vi "AB_1000_1100_Project_Build_Info.vi"(7 "action":T1, 8 "error in (no error)":errorcluster, 10 "buildInfo in":T2, 11 "Object In":T3) -> (0 "error out":errorcluster, 2 "buildInfo out":T2, 3 "Object Out":T3)   [LabVIEW 2020]
uses:
  <vilib>/AppBuilder/RW_Project/AB_RW_Project_PropBag_Action.ctl
  <resource>/Framework/Providers/API/ItemRef.ctl
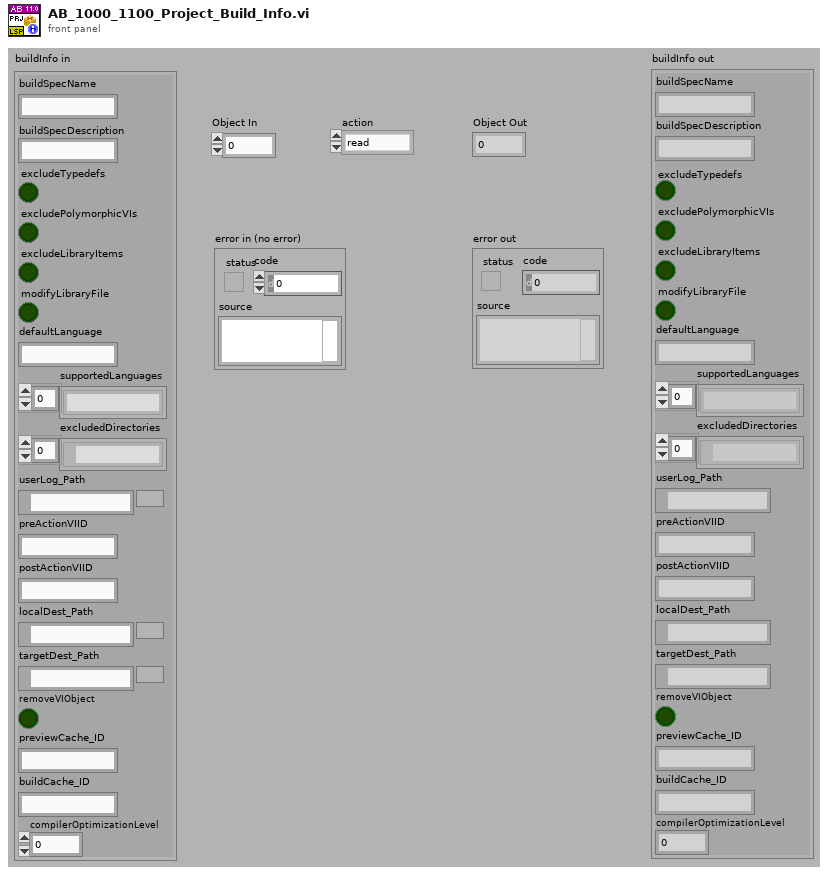
[diagram p1: front panel]
types:
  T1 = typedef "AB_RW_Project_PropBag_Action.ctl" = enum16{"read", "write", "clear", "readPrevious", "writePrevious", "clearPrevious"}
  T2 = cluster{"buildSpecName":string, "buildSpecDescription":string, "excludeTypedefs":bool, "excludePolymorphicVIs":bool, "excludeLibraryItems":bool, "modifyLibraryFile":bool, "defaultLanguage":string, "supportedLanguages":string[], "excludedDirectories":path[], "userLog_Path":path, "preActionVIID":string, "postActionVIID":string, "localDest_Path":path, "targetDest_Path":path, "removeVIObject":bool, "previewCache_ID":string, "buildCache_ID":string, "compilerOptimizationLevel":u32}
  T3 = typedef "ItemRef.ctl" = u64
  T4 = enum16{"<none>", "relativeToCommon", "relativeToAppDir"}
  T5 = typedef "AB_820_850_Relative_Path_Type.ctl" = enum16{"<none>", "relativeToCommon", "relativeToAppDir"}
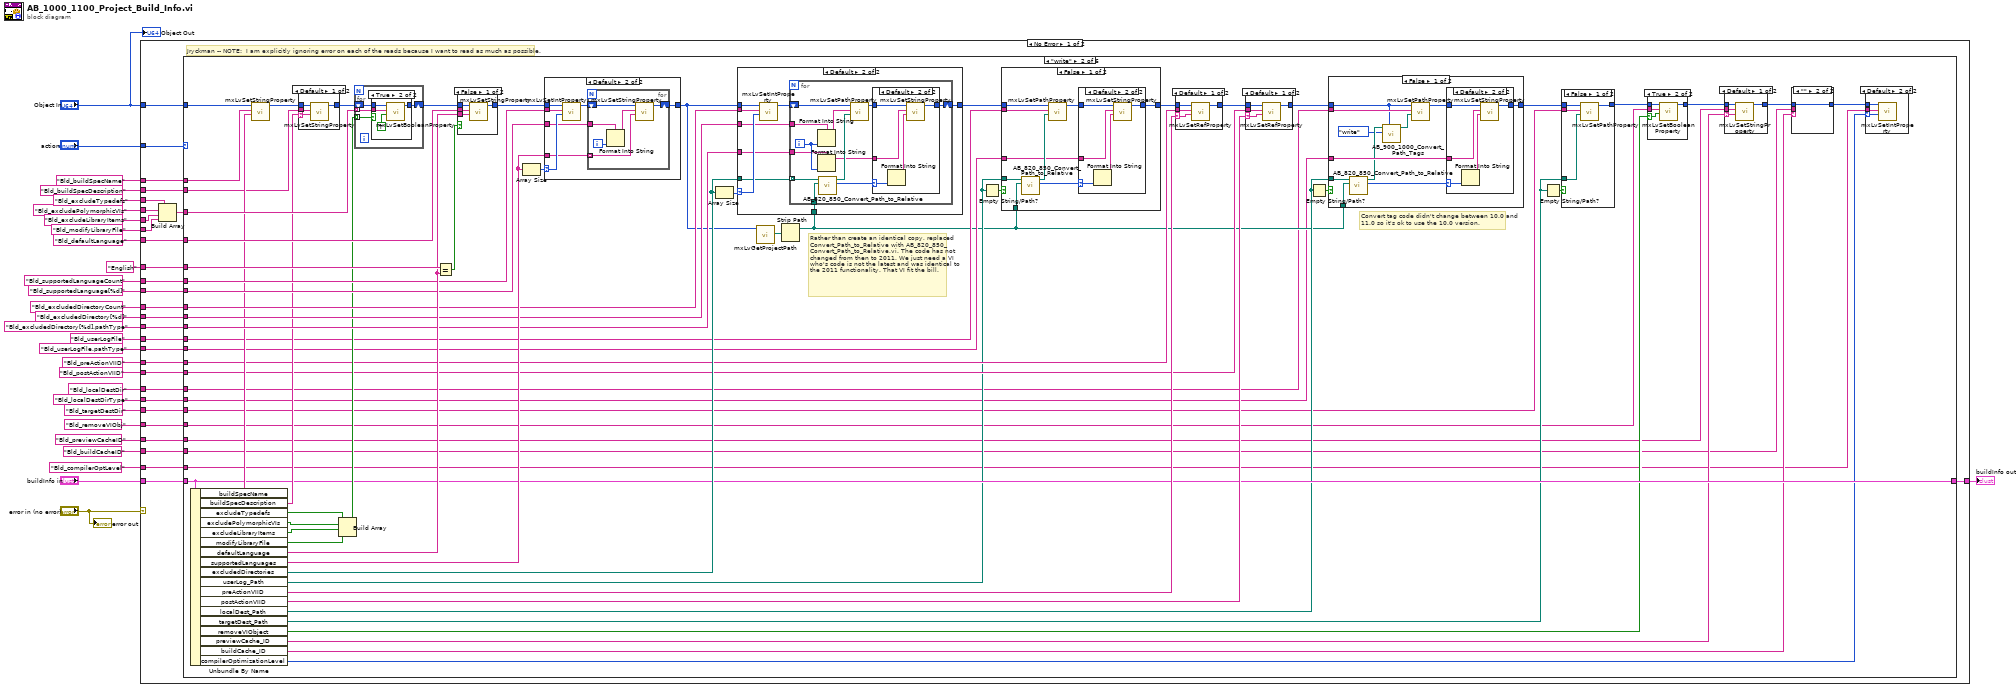
[diagram p0: block diagram]
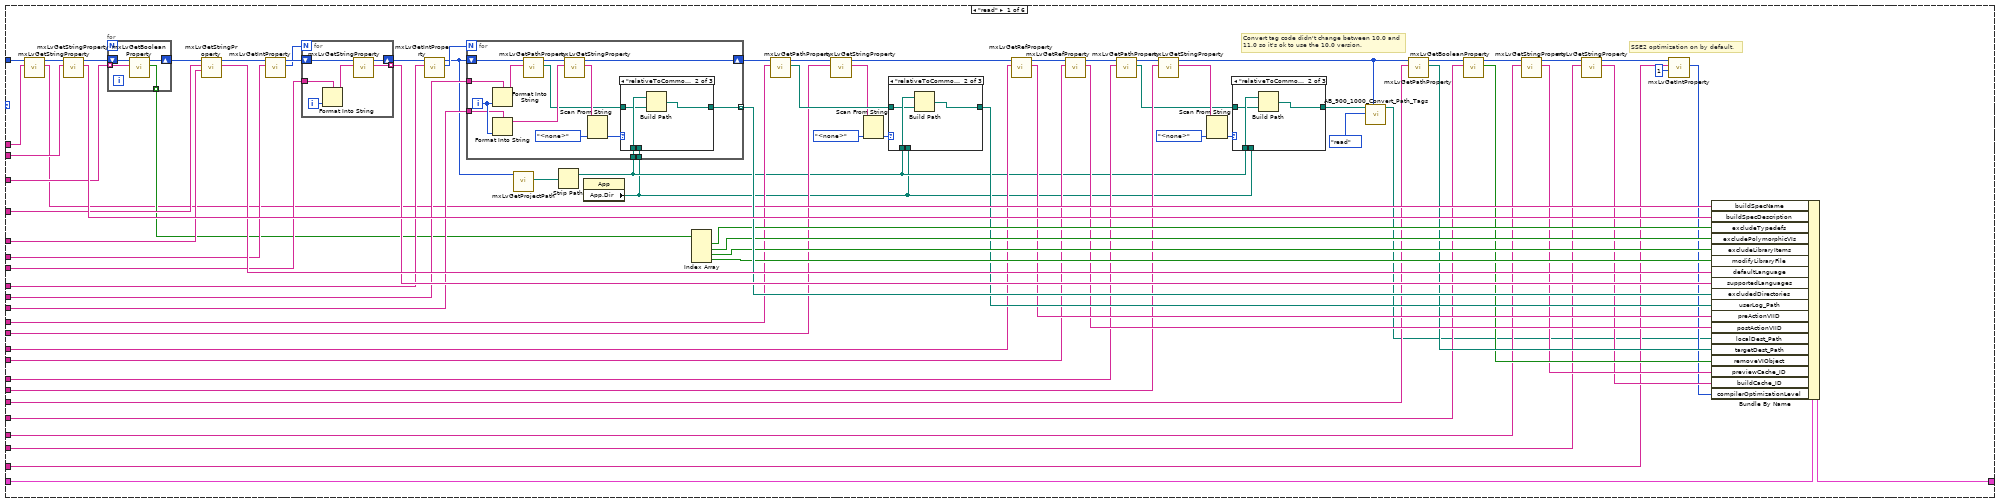
[diagram p2: hidden frame]
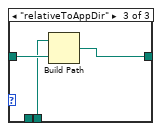
[diagram p4: hidden frame]
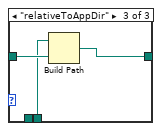
[diagram p6: hidden frame]
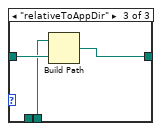
[diagram p8: hidden frame]
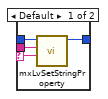
[diagram p10: hidden frame]
diagram:
  n1 = case shown="No Error" "error in (no error)" {
    tunnel: "Object In" -> [w58 _]
    tunnel: [w47 _] -> w27
    tunnel: "Bld_buildSpecDescription" ("Tag") -> [w57 _]
    tunnel: "Bld_excludeTypedefs" ("Tag") -> [w43 _]
    tunnel: "Bld_defaultLanguage" ("Tag") -> [w56 _]
    tunnel: "English" ("Tag") -> [w55 _]
    tunnel: "Bld_supportedLanguageCount" ("Tag") -> [w54 _]
    tunnel: "Bld_supportedLanguage[%d]" ("Tag") -> [w53 _]
    tunnel: "Bld_excludedDirectoryCount" ("Tag") -> [w52 _]
    tunnel: "Bld_excludedDirectory[%d]" ("Tag") -> [w51 _]
    tunnel: "Bld_excludedDirectory[%d].pathType" ("Tag") -> [w50 _]
    tunnel: "buildInfo in" -> [w49 _]
    tunnel: "action" -> [w48 _]
    tunnel: "Bld_excludePolymorphicVIs" ("Tag") -> [w46 _]
    tunnel: "Bld_excludeLibraryItems" ("Tag") -> [w45 _]
    tunnel: "Bld_modifyLibraryFile" ("Tag") -> [w44 _]
    tunnel: "Bld_buildSpecName" ("Tag") -> [w41 _]
    tunnel: "Bld_userLogFile" ("Tag") -> [w40 _]
    tunnel: "Bld_userLogFile.pathType" ("Tag") -> [w39 _]
    tunnel: "Bld_preActionVIID" ("Tag") -> [w38 _]
    tunnel: "Bld_postActionVIID" ("Tag") -> [w37 _]
    tunnel: "Bld_localDestDir" ("Tag") -> [w36 _]
    tunnel: "Bld_targetDestDir" ("Tag") -> [w35 _]
    tunnel: "Bld_localDestDirType" ("Tag") -> [w34 _]
    tunnel: "Bld_removeVIObj" ("Tag") -> [w33 _]
    tunnel: "Bld_previewCacheID" ("Tag") -> [w32 _]
    tunnel: "Bld_buildCacheID" ("Tag") -> [w31 _]
    tunnel: "Bld_compilerOptLevel" ("Tag") -> [w30 _]
    frame No Error {
      # "Jryckman -- NOTE:  I am explicitly ignoring error on each of the reads because I want to read as much as possible."
      n2 = Build Array(w43, w46, w45, w44) -> (w42:string[])
      n3 = case shown="\"write\"" w48 {
        tunnel: w58 -> [w108 w224 w411 _ w435 _]
        tunnel: w57 -> [w135 w219 w413 _ _ _]
        tunnel: w56 -> [w133 w244 w412 _ _ _]
        tunnel: w55 -> [w132 w243 _ _ _ _]
        tunnel: w54 -> [w129 w238 w410 _ _ _]
        tunnel: w53 -> [w126 w237 w407 _ _ _]
        tunnel: w52 -> [w123 w233 w403 _ _ _]
        tunnel: w51 -> [w121 w232 w402 _ _ _]
        tunnel: w50 -> [w120 w231 w401 _ _ _]
        tunnel: w49 -> [w117 w203 w398 w430 w436 w439]
        tunnel: [w118 w203 w398 w430 w436 w439] -> w47
        tunnel: w42 -> [w114 w225 w397 _ _ _]
        tunnel: w41 -> [w106 w222 w396 _ _ _]
        tunnel: w40 -> [w101 w216 w394 _ _ _]
        tunnel: w39 -> [w94 w212 w392 _ _ _]
        tunnel: w38 -> [w93 w210 w389 _ _ _]
        tunnel: w37 -> [w90 w207 w388 _ _ _]
        tunnel: w36 -> [w82 w198 w385 _ _ _]
        tunnel: w35 -> [w77 w196 w383 _ _ _]
        tunnel: w34 -> [w81 w199 w384 _ _ _]
        tunnel: w33 -> [w73 w192 w380 _ _ _]
        tunnel: w32 -> [w71 w189 w378 _ w433 _]
        tunnel: w31 -> [w68 w186 w376 _ w434 _]
        tunnel: w30 -> [w64 w182 w374 _ w431 _]
        frame "read" {
          # "Convert tag code didn't change between 10.0 and 11.0 so it's ok to use the 10.0 version."
          # "SSE2 optimization on by default."
          n4 = call <resource>:"mxLvGetStringProperty.vi"("Tag"=w106, "Item"=w108) -> ("Value"=w105:string, "Item"=w107:T3)  [unwired: 1 in, 7 out]
          n5 = call <resource>:"mxLvGetStringProperty.vi"("Tag"=w135, "Item"=w107) -> ("Value"=w134:string, "Item"=w116:T3)  [unwired: 1 in, 7 out]
          n6 = for {
            shift-right: [w153] -> w115
            shift-left: w116 -> [w151]
            tunnel: w114 -> [w152] mode=indexing
            tunnel: [w150] -> w113 mode=indexing
            n7 = call <resource>:"mxLvGetBooleanProperty.vi"("Tag"=w152, "Item"=w151) -> ("Value"=w150:bool, "Item"=w153:T3)  [unwired: 1 in, 7 out]
          }
          n8 = call <resource>:"mxLvGetStringProperty.vi"("Default Value (\"\")"=w132, "Tag"=w133, "Item"=w115) -> ("Value"=w131:string, "Item"=w130:T3)  [unwired: 1 in, 6 out]
          n9 = call <resource>:"mxLvGetIntProperty.vi"("Tag"=w129, "Item"=w130) -> ("Value"=w127:i32, "Item"=w128:T3)  [unwired: 1 in, 7 out]
          n10 = for {
            N: w127 -> [_]
            shift-right: [w178] -> w124
            shift-left: w128 -> [w179]
            tunnel: w126 -> [w180]
            tunnel: [w176] -> w125 mode=indexing
            i -> [w181]
            n11 = Format Into String(format string=w180, w181) -> (resulting string=w177:string)  [unwired: 2 in, 1 out]
            n12 = call <resource>:"mxLvGetStringProperty.vi"("Tag"=w177, "Item"=w179) -> ("Value"=w176:string, "Item"=w178:T3)  [unwired: 1 in, 7 out]
          }
          n13 = call <resource>:"mxLvGetIntProperty.vi"("Tag"=w123, "Item"=w124) -> ("Value"=w122:i32, "Item"=w104:T3)  [unwired: 1 in, 7 out]
          n14 = call <resource>:"mxLvGetProjectPath.vi"("Item"=w104) -> ("Project Path"=w103:path)  [unwired: 1 in, 9 out]
          n15 = Strip Path(path=w103) -> (stripped path=w79:path)  [unwired: 1 out]
          n16 = property class="App"() -> ("App.Dir"=w78:path)  [unwired: 2 in, 2 out]
          n17 = for {
            N: w122 -> [_]
            shift-right: [w155] -> w102
            shift-left: w104 -> [w165]
            tunnel: w121 -> [w168]
            tunnel: w120 -> [w166]
            tunnel: w79 -> [w158]
            tunnel: [w156] -> w119 mode=indexing
            tunnel: w78 -> [w154]
            i -> [w167]
            n18 = Format Into String(format string=w168, w167) -> (resulting string=w164:string)  [unwired: 2 in, 1 out]
            n19 = Format Into String(format string=w166, w167) -> (resulting string=w162:string)  [unwired: 2 in, 1 out]
            n20 = call <resource>:"mxLvGetPathProperty.vi"("Tag"=w164, "Item"=w165) -> ("Path"=w157:path, "Item"=w163:T3)  [unwired: 2 in, 6 out]
            n21 = call <resource>:"mxLvGetStringProperty.vi"("Tag"=w162, "Item"=w163) -> ("Value"=w161:string, "Item"=w155:T3)  [unwired: 1 in, 7 out]
            n22 = Scan From String(input string=w161, default 1=T4."<none>" ("relativeType")) -> (output 1=w159:T4)  [unwired: 3 in, 3 out]
            n23 = case shown="\"relativeToCommon\"" w159 {
              tunnel: w158 -> [_ w172 _]
              tunnel: w157 -> [w169 w171 w175]
              tunnel: [w169 w170 w174] -> w156
              tunnel: w154 -> [_ _ w173]
              frame "<none>" {
              }
              frame "relativeToCommon" {
                n24 = Build Path(base path=w172, name or relative path=w171) -> (appended path=w170:path)
              }
              frame "relativeToAppDir" {
                n25 = Build Path(base path=w173, name or relative path=w175) -> (appended path=w174:path)
              }
            }
          }
          n26 = Index Array(array=w113) -> (element #1=w112:bool, element #2=w111:bool, element #3=w110:bool, element #4=w109:bool)  [unwired: 4 in]
          n27 = call <resource>:"mxLvGetPathProperty.vi"("Tag"=w101, "Item"=w102) -> ("Path"=w98:path, "Item"=w96:T3)  [unwired: 2 in, 6 out]
          n28 = call <resource>:"mxLvGetStringProperty.vi"("Tag"=w94, "Item"=w96) -> ("Value"=w95:string, "Item"=w92:T3)  [unwired: 1 in, 7 out]
          n29 = Scan From String(input string=w95, default 1=T4."<none>" ("relativeType")) -> (output 1=w100:T4)  [unwired: 3 in, 3 out]
          n30 = case shown="\"relativeToCommon\"" w100 {
            tunnel: w79 -> [_ w146 _]
            tunnel: w98 -> [w143 w145 w149]
            tunnel: [w143 w144 w148] -> w97
            tunnel: w78 -> [_ _ w147]
            frame "<none>" {
            }
            frame "relativeToCommon" {
              n31 = Build Path(base path=w146, name or relative path=w145) -> (appended path=w144:path)
            }
            frame "relativeToAppDir" {
              n32 = Build Path(base path=w147, name or relative path=w149) -> (appended path=w148:path)
            }
          }
          n33 = call <resource>:"mxLvGetRefProperty.vi"("Tag"=w93, "Item"=w92) -> ("Value"=w91:string, "Item"=w89:T3)  [unwired: 1 in, 7 out]
          n34 = call <resource>:"mxLvGetRefProperty.vi"("Tag"=w90, "Item"=w89) -> ("Value"=w88:string, "Item"=w83:T3)  [unwired: 1 in, 7 out]
          n35 = call <resource>:"mxLvGetPathProperty.vi"("Tag"=w82, "Item"=w83) -> ("Path"=w80:path, "Item"=w84:T3)  [unwired: 2 in, 6 out]
          n36 = call <resource>:"mxLvGetStringProperty.vi"("Tag"=w81, "Item"=w84) -> ("Value"=w87:string, "Item"=w60:T3)  [unwired: 1 in, 7 out]
          n37 = Scan From String(input string=w87, default 1=T4."<none>" ("relativeType")) -> (output 1=w85:T4)  [unwired: 3 in, 3 out]
          n38 = case shown="\"relativeToCommon\"" w85 {
            tunnel: w79 -> [_ w139 _]
            tunnel: w80 -> [w136 w138 w142]
            tunnel: [w136 w137 w141] -> w61
            tunnel: w78 -> [_ _ w140]
            frame "<none>" {
            }
            frame "relativeToCommon" {
              n39 = Build Path(base path=w139, name or relative path=w138) -> (appended path=w137:path)
            }
            frame "relativeToAppDir" {
              n40 = Build Path(base path=w140, name or relative path=w142) -> (appended path=w141:path)
            }
          }
          n41 = call <vilib>:"AB_900_1000_Convert_Path_Tags.vi"("buildObject"=w60, "action"=AB_RW_Project_PropBag_Action."read", "Path in"=w61) -> ("Path out"=w62:path)  [unwired: 7 in, 1 out]
          n42 = call <resource>:"mxLvGetPathProperty.vi"("Tag"=w77, "Item"=w60) -> ("Path"=w76:path, "Item"=w75:T3)  [unwired: 2 in, 6 out]
          n43 = call <resource>:"mxLvGetBooleanProperty.vi"("Tag"=w73, "Item"=w75) -> ("Value"=w74:bool, "Item"=w72:T3)  [unwired: 1 in, 7 out]
          n44 = call <resource>:"mxLvGetStringProperty.vi"("Tag"=w71, "Item"=w72) -> ("Value"=w70:string, "Item"=w69:T3)  [unwired: 1 in, 7 out]
          n45 = call <resource>:"mxLvGetStringProperty.vi"("Tag"=w68, "Item"=w69) -> ("Value"=w67:string, "Item"=w66:T3)  [unwired: 1 in, 7 out]
          n46 = call <resource>:"mxLvGetIntProperty.vi"("Default Value (0)"=1, "Tag"=w64, "Item"=w66) -> ("Value"=w65:i32)  [unwired: 1 in, 7 out]
          n47 = Bundle By Name(cluster=w117, "buildSpecName"=w105, "buildSpecDescription"=w134, "excludeTypedefs"=w112, "excludePolymorphicVIs"=w111, "excludeLibraryItems"=w110, "modifyLibraryFile"=w109, "defaultLanguage"=w131, "supportedLanguages"=w125, "excludedDirectories"=w119, "userLog_Path"=w97, "preActionVIID"=w91, "postActionVIID"=w88, "localDest_Path"=w62, "targetDest_Path"=w76, "removeVIObject"=w74, "previewCache_ID"=w70, "buildCache_ID"=w67, "compilerOptimizationLevel"=w65) -> (w118:T2)
        }
        frame "write" {
          # "Convert tag code didn't change between 10.0 and 11.0 so it's ok to use the 10.0 version."
          # "Rather than create an identical copy, replaced  Convert_Path_to_Relative with AB_820_850_Convert_Path_to_Relative.vi. The code has not changed from then to 2011. We just need a VI who's code is not the latest and was identical to the 2011 functionality. That VI fit the bill."
          n48 = Unbundle By Name(w203) -> ("buildSpecName"=w223:string, "buildSpecDescription"=w218:string, "excludeTypedefs"=w230:bool, "excludePolymorphicVIs"=w229:bool, "excludeLibraryItems"=w228:bool, "modifyLibraryFile"=w227:bool, "defaultLanguage"=w242:string, "supportedLanguages"=w236:string[], "excludedDirectories"=w234:path[], "userLog_Path"=w202:path, "preActionVIID"=w209:string, "postActionVIID"=w206:string, "localDest_Path"=w201:path, "targetDest_Path"=w195:path, "removeVIObject"=w191:bool, "previewCache_ID"=w188:string, "buildCache_ID"=w185:string, "compilerOptimizationLevel"=w183:u32)
          n49 = call <resource>:"mxLvSetStringProperty.vi"("Value (\"\")"=w223, "Tag"=w222, "Item"=w224) -> ("Item"=w221:T3)  [unwired: 2 in, 6 out]
          n50 = case shown="Default" w218 {
            selector: w218 -> [w313 _]
            tunnel: w221 -> [w316 w317]
            tunnel: w219 -> [w315 _]
            tunnel: [w314 w317] -> w220
            frame Default {
              n51 = call <resource>:"mxLvSetStringProperty.vi"("Value (\"\")"=w313, "Tag"=w315, "Item"=w316) -> ("Item"=w314:T3)  [unwired: 2 in, 6 out]
            }
            frame "" {
            }
          }
          n52 = Build Array(w230, w229, w228, w227) -> (w226:bool[])
          n53 = for {
            shift-right: [w320] -> w245
            shift-left: w220 -> [w321]
            tunnel: w226 -> [w319] mode=indexing
            tunnel: w225 -> [w318] mode=indexing
            n54 = case shown="True" w319 {
              tunnel: w321 -> [w322 w326]
              tunnel: [w322 w325] -> w320
              tunnel: w318 -> [_ w324]
              frame False {
              }
              frame True {
                n55 = call <resource>:"mxLvSetBooleanProperty.vi"("Value (F)"=TRUE, "Tag"=w324, "Item"=w326) -> ("Item"=w325:T3)  [unwired: 2 in, 6 out]
              }
            }
          }
          n56 = Equal?(x=w243, y=w242) -> (x = y?=w241:bool)
          n57 = case shown="False" w241 {
            tunnel: w245 -> [w372 w373]
            tunnel: w244 -> [w371 _]
            tunnel: w242 -> [w370 _]
            tunnel: [w369 w373] -> w239
            frame False {
              n58 = call <resource>:"mxLvSetStringProperty.vi"("Value (\"\")"=w370, "Tag"=w371, "Item"=w372) -> ("Item"=w369:T3)  [unwired: 2 in, 6 out]
            }
            frame True {
            }
          }
          n59 = Array Size(array=w236) -> (size(s)=w240:i32)
          n60 = case shown="Default" w240 {
            selector: w240 -> [_ w360]
            tunnel: w239 -> [w355 w362]
            tunnel: w238 -> [_ w361]
            tunnel: w237 -> [_ w358]
            tunnel: w236 -> [_ w357]
            tunnel: [w355 w356] -> w213
            frame 0 {
            }
            frame Default {
              n61 = call <resource>:"mxLvSetIntProperty.vi"("Value (0)"=w360, "Tag"=w361, "Item"=w362) -> ("Item"=w359:T3)  [unwired: 2 in, 6 out]
              n62 = for {
                shift-right: [w367] -> w356
                shift-left: w359 -> [w368]
                tunnel: w358 -> [w365]
                tunnel: w357 -> [w363] mode=indexing
                i -> [w366]
                n63 = Format Into String(format string=w365, w366) -> (resulting string=w364:string)  [unwired: 2 in, 1 out]
                n64 = call <resource>:"mxLvSetStringProperty.vi"("Value (\"\")"=w363, "Tag"=w364, "Item"=w368) -> ("Item"=w367:T3)  [unwired: 2 in, 6 out]
              }
            }
          }
          n65 = Array Size(array=w234) -> (size(s)=w235:i32)
          n66 = call <resource>:"mxLvGetProjectPath.vi"("Item"=w213) -> ("Project Path"=w214:path)  [unwired: 1 in, 9 out]
          n67 = Strip Path(path=w214) -> (stripped path=w200:path)  [unwired: 1 out]
          n68 = case shown="Default" w235 {
            selector: w235 -> [_ w335]
            tunnel: w213 -> [w327 w330]
            tunnel: w233 -> [_ w336]
            tunnel: w232 -> [_ w333]
            tunnel: w234 -> [_ w332]
            tunnel: w231 -> [_ w331]
            tunnel: [w327 w329] -> w217
            tunnel: w200 -> [_ w328]
            frame 0 {
            }
            frame Default {
              n69 = call <resource>:"mxLvSetIntProperty.vi"("Value (0)"=w335, "Tag"=w336, "Item"=w330) -> ("Item"=w334:T3)  [unwired: 2 in, 6 out]
              n70 = for {
                shift-right: [w348] -> w329
                shift-left: w334 -> [w344]
                tunnel: w333 -> [w347]
                tunnel: w332 -> [w346] mode=indexing
                tunnel: w328 -> [w338]
                tunnel: w331 -> [w337]
                i -> [w342]
                n71 = Format Into String(format string=w347, w342) -> (resulting string=w345:string)  [unwired: 2 in, 1 out]
                n72 = Format Into String(format string=w337, w342) -> (resulting string=w340:string)  [unwired: 2 in, 1 out]
                n73 = call <vilib>:"AB_820_850_Convert_Path_to_Relative.vi"("commonPath"=w338, "absolutePath"=w346) -> ("relativeType"=w339:T5, "newPath"=w341:path)  [unwired: 7 in, 1 out]
                n74 = call <resource>:"mxLvSetPathProperty.vi"("Path"=w341, "Tag"=w345, "Item"=w344) -> ("Item"=w343:T3)  [unwired: 2 in, 6 out]
                n75 = case shown="Default" w339 {
                  selector: w339 -> [_ w350]
                  tunnel: [w349 w354] -> w348
                  tunnel: w343 -> [w349 w353]
                  tunnel: w340 -> [_ w351]
                  frame "<none>" {
                  }
                  frame Default {
                    n76 = Format Into String(w350) -> (resulting string=w352:string)  [unwired: 3 in, 1 out]
                    n77 = call <resource>:"mxLvSetStringProperty.vi"("Value (\"\")"=w352, "Tag"=w351, "Item"=w353) -> ("Item"=w354:T3)  [unwired: 2 in, 6 out]
                  }
                }
              }
            }
          }
          n78 = Empty String/Path?(string/path=w202) -> (empty?=w215:bool)
          n79 = case shown="False" w215 {
            tunnel: w217 -> [w305 w312]
            tunnel: w216 -> [w304 _]
            tunnel: w200 -> [w301 _]
            tunnel: w202 -> [w300 _]
            tunnel: w212 -> [w298 _]
            tunnel: [w297 w312] -> w211
            frame False {
              n80 = call <vilib>:"AB_820_850_Convert_Path_to_Relative.vi"("commonPath"=w301, "absolutePath"=w300) -> ("relativeType"=w303:T5, "newPath"=w299:path)  [unwired: 7 in, 1 out]
              n81 = call <resource>:"mxLvSetPathProperty.vi"("Path"=w299, "Tag"=w304, "Item"=w305) -> ("Item"=w302:T3)  [unwired: 2 in, 6 out]
              n82 = case shown="Default" w303 {
                selector: w303 -> [_ w308]
                tunnel: w302 -> [w306 w311]
                tunnel: w298 -> [_ w309]
                tunnel: [w306 w307] -> w297
                frame "<none>" {
                }
                frame Default {
                  n83 = Format Into String(w308) -> (resulting string=w310:string)  [unwired: 3 in, 1 out]
                  n84 = call <resource>:"mxLvSetStringProperty.vi"("Value (\"\")"=w310, "Tag"=w309, "Item"=w311) -> ("Item"=w307:T3)  [unwired: 2 in, 6 out]
                }
              }
            }
            frame True {
            }
          }
          n85 = case shown="Default" w209 {
            selector: w209 -> [w293 _]
            tunnel: w211 -> [w295 w296]
            tunnel: w210 -> [w294 _]
            tunnel: [w292 w296] -> w208
            frame Default {
              n86 = call <resource>:"mxLvSetRefProperty.vi"("Value (\"\")"=w293, "Tag"=w294, "Item"=w295) -> ("Item"=w292:T3)  [unwired: 2 in, 6 out]
            }
            frame "" {
            }
          }
          n87 = case shown="Default" w206 {
            selector: w206 -> [w288 _]
            tunnel: w208 -> [w290 w291]
            tunnel: w207 -> [w289 _]
            tunnel: [w287 w291] -> w204
            frame Default {
              n88 = call <resource>:"mxLvSetRefProperty.vi"("Value (\"\")"=w288, "Tag"=w289, "Item"=w290) -> ("Item"=w287:T3)  [unwired: 2 in, 6 out]
            }
            frame "" {
            }
          }
          n89 = Empty String/Path?(string/path=w201) -> (empty?=w205:bool)
          n90 = case shown="False" w205 {
            tunnel: w204 -> [w269 w286]
            tunnel: w198 -> [w279 _]
            tunnel: w200 -> [w276 _]
            tunnel: w201 -> [w275 _]
            tunnel: w199 -> [w274 _]
            tunnel: [w273 w286] -> w197
            frame False {
              n91 = call <vilib>:"AB_820_850_Convert_Path_to_Relative.vi"("commonPath"=w276, "absolutePath"=w275) -> ("relativeType"=w278:T5, "newPath"=w272:path)  [unwired: 7 in, 1 out]
              n92 = call <vilib>:"AB_900_1000_Convert_Path_Tags.vi"("buildObject"=w269, "action"=AB_RW_Project_PropBag_Action."write", "Path in"=w272) -> ("Path out"=w271:path)  [unwired: 7 in, 1 out]
              n93 = call <resource>:"mxLvSetPathProperty.vi"("Path"=w271, "Tag"=w279, "Item"=w269) -> ("Item"=w277:T3)  [unwired: 2 in, 6 out]
              n94 = case shown="Default" w278 {
                selector: w278 -> [_ w282]
                tunnel: w277 -> [w280 w285]
                tunnel: w274 -> [_ w283]
                tunnel: [w280 w281] -> w273
                frame "<none>" {
                }
                frame Default {
                  n95 = Format Into String(w282) -> (resulting string=w284:string)  [unwired: 3 in, 1 out]
                  n96 = call <resource>:"mxLvSetStringProperty.vi"("Value (\"\")"=w284, "Tag"=w283, "Item"=w285) -> ("Item"=w281:T3)  [unwired: 2 in, 6 out]
                }
              }
            }
            frame True {
            }
          }
          n97 = Empty String/Path?(string/path=w195) -> (empty?=w194:bool)
          n98 = case shown="False" w194 {
            tunnel: w197 -> [w267 w268]
            tunnel: w196 -> [w266 _]
            tunnel: w195 -> [w265 _]
            tunnel: [w264 w268] -> w193
            frame False {
              n99 = call <resource>:"mxLvSetPathProperty.vi"("Path"=w265, "Tag"=w266, "Item"=w267) -> ("Item"=w264:T3)  [unwired: 2 in, 6 out]
            }
            frame True {
            }
          }
          n100 = case shown="True" w191 {
            selector: w191 -> [_ w261]
            tunnel: w193 -> [w259 w263]
            tunnel: w192 -> [_ w262]
            tunnel: [w259 w260] -> w190
            frame False {
            }
            frame True {
              n101 = call <resource>:"mxLvSetBooleanProperty.vi"("Value (F)"=w261, "Tag"=w262, "Item"=w263) -> ("Item"=w260:T3)  [unwired: 2 in, 6 out]
            }
          }
          n102 = case shown="Default" w188 {
            selector: w188 -> [w255 _]
            tunnel: w190 -> [w257 w258]
            tunnel: w189 -> [w256 _]
            tunnel: [w254 w258] -> w187
            frame Default {
              n103 = call <resource>:"mxLvSetStringProperty.vi"("Value (\"\")"=w255, "Tag"=w256, "Item"=w257) -> ("Item"=w254:T3)  [unwired: 2 in, 6 out]
            }
            frame "" {
            }
          }
          n104 = case shown="\"\"" w185 {
            selector: w185 -> [w250 _]
            tunnel: w187 -> [w252 w253]
            tunnel: w186 -> [w251 _]
            tunnel: [w249 w253] -> w184
            frame Default {
              n105 = call <resource>:"mxLvSetStringProperty.vi"("Value (\"\")"=w250, "Tag"=w251, "Item"=w252) -> ("Item"=w249:T3)  [unwired: 2 in, 6 out]
            }
            frame "" {
            }
          }
          n106 = case shown="Default" w183 {
            selector: w183 -> [_ w247]
            tunnel: w184 -> [_ w248]
            tunnel: w182 -> [_ w246]
            frame 1 {
            }
            frame Default {
              n107 = call <resource>:"mxLvSetIntProperty.vi"("Value (0)"=w247, "Tag"=w246, "Item"=w248) -> ()  [unwired: 2 in, 7 out]
            }
          }
        }
        frame "clear" {
          n108 = Build Array (concatenate)(w396, w413, w397, w412, w410, w403) -> (w399:string[])
          n109 = call <resource>:"mxLvGetIntProperty.vi"("Tag"=w410, "Item"=w411) -> ("Value"=w408:i32, "Item"=w409:T3)  [unwired: 1 in, 7 out]
          n110 = for {
            N: w408 -> [_]
            shift-right: [w426] -> w404
            shift-left: w409 -> [w427]
            tunnel: w407 -> [w428]
            i -> [w429]
            n111 = Format Into String(format string=w428, w429) -> (resulting string=w425:string)  [unwired: 2 in, 1 out]
            n112 = call <resource>:"mxLvDeleteProperty.vi"("Tag"=w425, "Item"=w427) -> ("Item"=w426:T3)  [unwired: 1 in, 8 out]
          }
          n113 = call <resource>:"mxLvGetIntProperty.vi"("Tag"=w403, "Item"=w404) -> ("Value"=w406:i32, "Item"=w405:T3)  [unwired: 1 in, 7 out]
          n114 = for {
            N: w406 -> [_]
            shift-right: [w420] -> w400
            shift-left: w405 -> [w423]
            tunnel: w402 -> [w424]
            tunnel: w401 -> [w418]
            i -> [w419]
            n115 = Format Into String(format string=w424, w419) -> (resulting string=w422:string)  [unwired: 2 in, 1 out]
            n116 = Format Into String(format string=w418, w419) -> (resulting string=w417:string)  [unwired: 2 in, 1 out]
            n117 = call <resource>:"mxLvDeleteProperty.vi"("Tag"=w422, "Item"=w423) -> ("Item"=w421:T3)  [unwired: 1 in, 8 out]
            n118 = call <resource>:"mxLvDeleteProperty.vi"("Tag"=w417, "Item"=w421) -> ("Item"=w420:T3)  [unwired: 1 in, 8 out]
          }
          n119 = for {
            tunnel: w399 -> [w415] mode=indexing
            shift-right: [w414] -> w395
            shift-left: w400 -> [w416]
            n120 = call <resource>:"mxLvDeleteProperty.vi"("Tag"=w415, "Item"=w416) -> ("Item"=w414:T3)  [unwired: 1 in, 8 out]
          }
          n121 = call <resource>:"mxLvDeleteProperty.vi"("Tag"=w394, "Item"=w395) -> ("Item"=w393:T3)  [unwired: 1 in, 8 out]
          n122 = call <resource>:"mxLvDeleteProperty.vi"("Tag"=w392, "Item"=w393) -> ("Item"=w390:T3)  [unwired: 1 in, 8 out]
          n123 = call <resource>:"mxLvDeleteProperty.vi"("Tag"=w389, "Item"=w390) -> ("Item"=w391:T3)  [unwired: 1 in, 8 out]
          n124 = call <resource>:"mxLvDeleteProperty.vi"("Tag"=w388, "Item"=w391) -> ("Item"=w382:T3)  [unwired: 1 in, 8 out]
          n125 = call <resource>:"mxLvDeleteProperty.vi"("Tag"=w385, "Item"=w382) -> ("Item"=w387:T3)  [unwired: 1 in, 8 out]
          n126 = call <resource>:"mxLvDeleteProperty.vi"("Tag"=w384, "Item"=w387) -> ("Item"=w386:T3)  [unwired: 1 in, 8 out]
          n127 = call <resource>:"mxLvDeleteProperty.vi"("Tag"=w383, "Item"=w386) -> ("Item"=w381:T3)  [unwired: 1 in, 8 out]
          n128 = call <resource>:"mxLvDeleteProperty.vi"("Tag"=w380, "Item"=w381) -> ("Item"=w379:T3)  [unwired: 1 in, 8 out]
          n129 = call <resource>:"mxLvDeleteProperty.vi"("Tag"=w378, "Item"=w379) -> ("Item"=w377:T3)  [unwired: 1 in, 8 out]
          n130 = call <resource>:"mxLvDeleteProperty.vi"("Tag"=w376, "Item"=w377) -> ("Item"=w375:T3)  [unwired: 1 in, 8 out]
          n131 = call <resource>:"mxLvDeleteProperty.vi"("Tag"=w374, "Item"=w375) -> ()  [unwired: 1 in, 9 out]
        }
        frame "readPrevious" {
        }
        frame "writePrevious" {
          n132 = Build Array(w433, w434, w431) -> (w432:string[])
          n133 = for {
            tunnel: w435 -> [w438]
            tunnel: w432 -> [w437] mode=indexing
            n134 = call <resource>:"mxLvDeleteProperty.vi"("Tag"=w437, "Item"=w438) -> ()  [unwired: 1 in, 9 out]
          }
        }
        frame "clearPrevious" {
        }
      }
    }
    frame Error {
    }
  }
  "buildInfo out" <- w27
  "Object Out" <- "Object In"
  "error out" <- "error in (no error)"
